vi "Session merge.vi"(7 "Loop Data":T1={"Persistent"={"Last file"=path "", "Last user"="", "Users"=[]}, "Temp handle"={"Connected"=FALSE, "Temp ctrl"={"Gain (P)"=0.0, "Reset (I)"=0.0, "Rate (D)"=0.0, "Stabilization rate"=0.0, "Stabilization delta"=0.0, "Type"=enum."Lake Shore 325", "Custom temp ctrl"={"VISA resource name"=""}, "Lakeshore 325"={"VISA name"="", "Loop"=0, "Heater Range"=1, "Heater Resistance"=0, "Sample sensor"=0, "Fast sensor"=0, "Slow sensor"=0}, "Lakeshore 331"={"VISA name"="", "Loop"=1, "Heater Range"=0, "Sample sensor"=0, "Fast sensor"=0, "Slow sensor"=0}, "Lakeshore 332"={"VISA name"="", "Loop"=1, "Heater Range"=0, "Sample sensor"=0, "Fast sensor"=0, "Slow sensor"=0}, "Lakeshore 335"={"VISA name"="", "Loop"=1, "Sample sensor"=0, "Fast sensor"=0, "Slow sensor"=0}}}, "Paths"={"Manual"=path "", "Settings"=path "", "Persistent"=path "", "Work dir."=path ""}, "Settings"={"MFIA"={"Address"="", "Use compensation"=FALSE, "Shut down gracefully"=FALSE}, "Temp ctrl"={"Gain (P)"=0.0, "Reset (I)"=0.0, "Rate (D)"=0.0, "Stabilization rate"=0.0, "Stabilization delta"=0.0, "Type"=enum."Lake Shore 325", "Custom temp ctrl"={"VISA resource name"=""}, "Lakeshore 325"={"VISA name"="", "Loop"=0, "Heater Range"=1, "Heater Resistance"=0, "Sample sensor"=0, "Fast sensor"=0, "Slow sensor"=0}, "Lakeshore 331"={"VISA name"="", "Loop"=1, "Heater Range"=0, "Sample sensor"=0, "Fast sensor"=0, "Slow sensor"=0}, "Lakeshore 332"={"VISA name"="", "Loop"=1, "Heater Range"=0, "Sample sensor"=0, "Fast sensor"=0, "Slow sensor"=0}, "Lakeshore 335"={"VISA name"="", "Loop"=1, "Sample sensor"=0, "Fast sensor"=0, "Slow sensor"=0}}, "Source-meter"={"Type"=enum."Custom", "Custom source-meter"={"VISA resource name"=""}, "Keithley 2600"={"VISA name"=""}}, "Other"={"Enable OriginLab"=FALSE, "Reader mode"=FALSE, "Auto-save"=FALSE}, "Defaults"={"IV properties"={"T"=300.0, "Vstart"=-0.5, "Vstop"=0.5, "Vpoints"=10.0, "Settling"=0.01, "I limit"=0.1, "Log mapping"=FALSE, "Averaging"=0.0}, "CV properties"={"T"=0.0, "Vstart"=-0.5, "Vstop"=0.5, "Vpoints"=10.0, "Precision"=enum."Normal", "Test signal"=0.01, "Auto I range"=FALSE, "Test frequency"=1000000.0, "I range"=-2.0, "V range"=10.0, "Log mapping"=FALSE, "Rel perm"=0.0, "Area"=0.0}, "DLTS properties"={"Tstart"=100.0, "Instant start"=FALSE, "Tstop"=300.0, "T rate"=5.0, "Test signal"=0.1, "Test frequency"=1000000.0, "Bandwidth"=5000.0, "Averaging"=10.0, "Vbias"=-2.0, "Vpulse"=-1.0, "pulse length"=0.001, "Pulse 2"=FALSE, "Vpulse 2"=0.0, "pulse length 2"=0.0, "I range"=-2.0, "V range"=10.0, "Emission rate"=[], "Sampling rate"=107142.859375, "Acq. delay"=0.0002}, "LDLTS properties"={"T"=0.0, "Test signal"=0.0, "Test frequency"=0.0, "Bandwidth"=0.0, "Averaging"=0.0, "Vbias"=0.0, "Vpulse"=0.0, "pulse length"=0.0, "Pulse 2"=FALSE, "Vpulse 2"=0.0, "pulse length 2"=0.0, "I range"=-2.0, "V range"=10.0, "Sampling rate"=0.0, "Acq. delay"=0.0, "Sampling time"=0.0}}}, "Software version"=0.0, "MFIA handle"={"ziHandle"={"handleValid"=FALSE, "Conn"=0, "Path Prefix"="", "Handle"=0, "Connected"=FALSE, "Clockbase(s)"=0.0}, "Selected device"="", "ziModHandle"={"handleValid"=FALSE, "Conn"=0, "ModHandle"=0, "moduleID"="", "Path Prefix"=""}}, "Source-meter handle"={"Connected"=FALSE, "Source-meter"={"Type"=enum."Keithley 2600", "Custom source-meter"={"VISA resource name"=""}, "Keithley 2600"={"VISA name"=""}}}} {"MFIA handle"."ziModHandle"."ModHandle" format="0x%08x"; "MFIA handle"."ziModHandle"."Conn" format="0x%08x"; "MFIA handle"."ziHandle"."Handle" format="0x%08x"; "MFIA handle"."ziHandle"."Conn" format="0x%08x"; "Settings"."Defaults"."LDLTS properties"."V range" items=["10mV"=0.01, "100mV"=0.1, "1V"=1.0, "10V"=10.0]; "Settings"."Defaults"."LDLTS properties"."I range" items=["100nA"=-7.0, "1µA"=-6.0, "10µA"=-5.0, "100µA"=-4.0, "1mA"=-3.0, "10mA"=-2.0]; "Settings"."Defaults"."DLTS properties"."V range" items=["10mV"=0.01, "100mV"=0.1, "1V"=1.0, "10V"=10.0]; "Settings"."Defaults"."DLTS properties"."I range" items=["10mV"=0.01, "100mV"=0.1, "1V"=1.0, "10V"=10.0]; "Settings"."Defaults"."CV properties"."V range" items=["10mV"=0.01, "100mV"=0.1, "1V"=1.0, "10V"=10.0]; "Settings"."Defaults"."CV properties"."I range" items=["100nA"=-7.0, "1µA"=-6.0, "10µA"=-5.0, "100µA"=-4.0, "1mA"=-3.0, "10mA"=-2.0]; "Settings"."Defaults"."IV properties"."Settling" min=0.0 max=65535.0; "Settings"."Temp ctrl"."Lakeshore 335"."Slow sensor" items=["A", "B"]; "Settings"."Temp ctrl"."Lakeshore 335"."Fast sensor" items=["A", "B"]; "Settings"."Temp ctrl"."Lakeshore 335"."Sample sensor" items=["A", "B"]; "Settings"."Temp ctrl"."Lakeshore 335"."Loop" items=["Loop 1"=1, "Loop 2"=2]; "Settings"."Temp ctrl"."Lakeshore 332"."Slow sensor" items=["A", "B"]; "Settings"."Temp ctrl"."Lakeshore 332"."Fast sensor" items=["A", "B"]; "Settings"."Temp ctrl"."Lakeshore 332"."Sample sensor" items=["A", "B"]; "Settings"."Temp ctrl"."Lakeshore 332"."Heater Range" items=["Off", "Low (0.5W)", "Med (5W)", "High (50W)"]; "Settings"."Temp ctrl"."Lakeshore 332"."Loop" items=["Loop 1", "Loop 2"]; "Settings"."Temp ctrl"."Lakeshore 331"."Slow sensor" items=["A", "B"]; "Settings"."Temp ctrl"."Lakeshore 331"."Fast sensor" items=["A", "B"]; "Settings"."Temp ctrl"."Lakeshore 331"."Sample sensor" items=["A", "B"]; "Settings"."Temp ctrl"."Lakeshore 331"."Heater Range" items=["Off", "Low (0.5W)", "Med (5W)", "High (50W)"]; "Settings"."Temp ctrl"."Lakeshore 331"."Loop" items=["Loop 1", "Loop 2"]; "Settings"."Temp ctrl"."Lakeshore 325"."Slow sensor" items=["A", "B"]; "Settings"."Temp ctrl"."Lakeshore 325"."Fast sensor" items=["A", "B"]; "Settings"."Temp ctrl"."Lakeshore 325"."Sample sensor" items=["A", "B"]; "Settings"."Temp ctrl"."Lakeshore 325"."Heater Resistance" items=["25 Ohm"=1, "50 Ohm"=2]; "Settings"."Temp ctrl"."Lakeshore 325"."Heater Range" items=["Off", "Low (loop 1) or On (loop 2)", "High (loop 1)"]; "Settings"."Temp ctrl"."Lakeshore 325"."Loop" items=["Loop 1"=1, "Loop 2"=2]; "Temp handle"."Temp ctrl"."Lakeshore 335"."Slow sensor" items=["A", "B"]; "Temp handle"."Temp ctrl"."Lakeshore 335"."Fast sensor" items=["A", "B"]; "Temp handle"."Temp ctrl"."Lakeshore 335"."Sample sensor" items=["A", "B"]; "Temp handle"."Temp ctrl"."Lakeshore 335"."Loop" items=["Loop 1"=1, "Loop 2"=2]; "Temp handle"."Temp ctrl"."Lakeshore 332"."Slow sensor" items=["A", "B"]; "Temp handle"."Temp ctrl"."Lakeshore 332"."Fast sensor" items=["A", "B"]; "Temp handle"."Temp ctrl"."Lakeshore 332"."Sample sensor" items=["A", "B"]; "Temp handle"."Temp ctrl"."Lakeshore 332"."Heater Range" items=["Off", "Low (0.5W)", "Med (5W)", "High (50W)"]; "Temp handle"."Temp ctrl"."Lakeshore 332"."Loop" items=["Loop 1", "Loop 2"]; "Temp handle"."Temp ctrl"."Lakeshore 331"."Slow sensor" items=["A", "B"]; "Temp handle"."Temp ctrl"."Lakeshore 331"."Fast sensor" items=["A", "B"]; "Temp handle"."Temp ctrl"."Lakeshore 331"."Sample sensor" items=["A", "B"]; "Temp handle"."Temp ctrl"."Lakeshore 331"."Heater Range" items=["Off", "Low (0.5W)", "Med (5W)", "High (50W)"]; "Temp handle"."Temp ctrl"."Lakeshore 331"."Loop" items=["Loop 1", "Loop 2"]; "Temp handle"."Temp ctrl"."Lakeshore 325"."Slow sensor" items=["A", "B"]; "Temp handle"."Temp ctrl"."Lakeshore 325"."Fast sensor" items=["A", "B"]; "Temp handle"."Temp ctrl"."Lakeshore 325"."Sample sensor" items=["A", "B"]; "Temp handle"."Temp ctrl"."Lakeshore 325"."Heater Resistance" items=["25 Ohm"=1, "50 Ohm"=2]; "Temp handle"."Temp ctrl"."Lakeshore 325"."Heater Range" items=["Off", "Low (loop 1) or On (loop 2)", "High (loop 1)"]; "Temp handle"."Temp ctrl"."Lakeshore 325"."Loop" items=["Loop 1"=1, "Loop 2"=2]}, 8 "Error In":errorcluster, 9 "Workspace":path, 10 "Index In":T20 {"IV"."IV properties"."Settling" min=0.0 max=65535.0; "CV"."CV properties"."V range" items=["10mV"=0.01, "100mV"=0.1, "1V"=1.0, "10V"=10.0]; "CV"."CV properties"."I range" items=["100nA"=-7.0, "1µA"=-6.0, "10µA"=-5.0, "100µA"=-4.0, "1mA"=-3.0, "10mA"=-2.0]; "LDLTS"."LDLTS properties"."V range" items=["10mV"=0.01, "100mV"=0.1, "1V"=1.0, "10V"=10.0]; "LDLTS"."LDLTS properties"."I range" items=["100nA"=-7.0, "1µA"=-6.0, "10µA"=-5.0, "100µA"=-4.0, "1mA"=-3.0, "10mA"=-2.0]; "Conv DLTS"."DLTS properties"."V range" items=["10mV"=0.01, "100mV"=0.1, "1V"=1.0, "10V"=10.0]; "Conv DLTS"."DLTS properties"."I range" items=["10mV"=0.01, "100mV"=0.1, "1V"=1.0, "10V"=10.0]}, 11 "Session properties in":T25) -> (0 "Error Out":errorcluster, 1 "Imported measurements count":i32, 2 "Index Out":T20 {"IV"."IV properties"."Settling" min=0.0 max=65535.0; "CV"."CV properties"."V range" items=["10mV"=0.01, "100mV"=0.1, "1V"=1.0, "10V"=10.0]; "CV"."CV properties"."I range" items=["100nA"=-7.0, "1µA"=-6.0, "10µA"=-5.0, "100µA"=-4.0, "1mA"=-3.0, "10mA"=-2.0]; "LDLTS"."LDLTS properties"."V range" items=["10mV"=0.01, "100mV"=0.1, "1V"=1.0, "10V"=10.0]; "LDLTS"."LDLTS properties"."I range" items=["100nA"=-7.0, "1µA"=-6.0, "10µA"=-5.0, "100µA"=-4.0, "1mA"=-3.0, "10mA"=-2.0]; "Conv DLTS"."DLTS properties"."V range" items=["10mV"=0.01, "100mV"=0.1, "1V"=1.0, "10V"=10.0]; "Conv DLTS"."DLTS properties"."I range" items=["10mV"=0.01, "100mV"=0.1, "1V"=1.0, "10V"=10.0]}, 3 "Session properties out":T25)   [LabVIEW 2019]
doc: "Displays information about a session"
uses:
  Type defs/Session properties Type Def.ctl
  Type defs/Session internal index Type Def.ctl
  Type defs/IV measurement Type Def.ctl
  Type defs/IV properties Type Def.ctl
  Type defs/CV measurement Type Def.ctl
  Type defs/CV properties Type Def.ctl
  Type defs/LDLTS measurement Type Def.ctl
  Type defs/LDLTS properties Type Def.ctl
  Type defs/cDLTS measurement Type Def.ctl
  Type defs/DLTS properties Type Def.ctl
  Type defs/Loop data Type Def.ctl
  Type defs/Persistent Type Def.ctl
  Type defs/Temp handle Type Def.ctl
  Type defs/Temp ctrl Type Def.ctl
  Custom devices/Custom temp ctrl settings.ctl
  Type defs/Paths Type Def.ctl
  Type defs/Settings Type Def.ctl
  Type defs/Imps Type Def.ctl
  Type defs/Source-meter Type Def.ctl
  Custom devices/Custom source-meter settings.ctl
  Type defs/Other settings Type Def.ctl
  Type defs/MFIA handle Type Def.ctl
  <instrlib>/Zurich Instruments LabOne/Public/ziTypeHandle.ctl
  <instrlib>/Zurich Instruments LabOne/Public/Modules/ziTypeModHandle.ctl
  Type defs/Source-meter handle Type Def.ctl
  <instrlib>/Zurich Instruments LabOne/Zurich Instruments LabOne.lvlib
panel:
  in  "Listbox":i32[](listbox) caption="Select measurements to import (duplicates cannot be imported)"
  out "Comment 2":string caption="Comment"
  out "Session Name 2":string caption="You're importing:"
  in  "Restore comment":bool
  in  "Restore name":bool
  in  "Cancel":bool
  in  "Apply":bool
  in  "Comment 1":string caption="Comment of the primary session"
  in  "Session Name 1":string caption="into the current session named:"
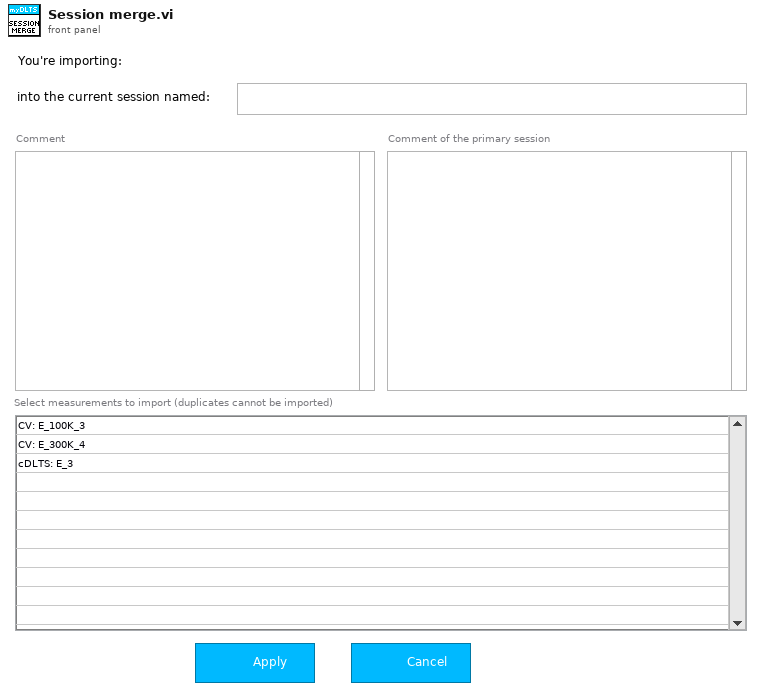
[diagram p1: front panel]
types:
  T1 = typedef "Loop data Type Def.ctl" = cluster{"Persistent":T2, "Temp handle":T3, "Paths":T6, "Settings":T7, "Software version":dbl, "MFIA handle":T16, "Source-meter handle":T19}
  T2 = typedef "Persistent Type Def.ctl" = cluster{"Last file":path, "Last user":string, "Users":cluster{"User":string, "Authors directory":path}[]}
  T3 = typedef "Temp handle Type Def.ctl" = cluster{"Connected":bool, "Temp ctrl":T4}
  T4 = typedef "Temp ctrl Type Def.ctl" = cluster{"Gain (P)":dbl, "Reset (I)":dbl, "Rate (D)":dbl, "Stabilization rate":dbl, "Stabilization delta":dbl, "Type":enum16{"Custom", "Lake Shore 325", "Lake Shore 331", "Lake Shore 332", "Lake Shore 335"}, "Custom temp ctrl":T5, "Lakeshore 325":cluster{"VISA name":refnum<visa-resource-name>, "Loop":u16, "Heater Range":u16, "Heater Resistance":u16, "Sample sensor":u16, "Fast sensor":u16, "Slow sensor":u16}, "Lakeshore 331":cluster{"VISA name":refnum<visa-resource-name>, "Loop":u16, "Heater Range":u16, "Sample sensor":u16, "Fast sensor":u16, "Slow sensor":u16}, "Lakeshore 332":cluster{"VISA name":refnum<visa-resource-name>, "Loop":u16, "Heater Range":u16, "Sample sensor":u16, "Fast sensor":u16, "Slow sensor":u16}, "Lakeshore 335":cluster{"VISA name":refnum<visa-resource-name>, "Loop":u16, "Sample sensor":u16, "Fast sensor":u16, "Slow sensor":u16}}
  T5 = typedef "Custom temp ctrl settings.ctl" = cluster{"VISA resource name":refnum<visa-resource-name>}
  T6 = typedef "Paths Type Def.ctl" = cluster{"Manual":path, "Settings":path, "Persistent":path, "Work dir.":path}
  T7 = typedef "Settings Type Def.ctl" = cluster{"MFIA":T8, "Temp ctrl":T4, "Source-meter":T9, "Other":T11, "Defaults":cluster{"IV properties":T12, "CV properties":T13, "DLTS properties":T14, "LDLTS properties":T15}}
  T8 = typedef "Imps Type Def.ctl" = cluster{"Address":string, "Use compensation":bool, "Shut down gracefully":bool}
  T9 = typedef "Source-meter Type Def.ctl" = cluster{"Type":enum16{"Custom", "Keithley 2600"}, "Custom source-meter":T10, "Keithley 2600":cluster{"VISA name":refnum<visa-resource-name>}}
  T10 = typedef "Custom source-meter settings.ctl" = cluster{"VISA resource name":refnum<visa-resource-name>}
  T11 = typedef "Other settings Type Def.ctl" = cluster{"Enable OriginLab":bool, "Reader mode":bool, "Auto-save":bool}
  T12 = typedef "IV properties Type Def.ctl" = cluster{"T":dbl[unit], "Vstart":dbl[unit], "Vstop":dbl[unit], "Vpoints":dbl, "Settling":dbl[unit], "I limit":dbl[unit], "Log mapping":bool, "Averaging":dbl}
  T13 = typedef "CV properties Type Def.ctl" = cluster{"T":dbl[unit], "Vstart":dbl[unit], "Vstop":dbl[unit], "Vpoints":dbl, "Precision":enum16{"Low (Fast)", "Normal", "High (Slow)"}, "Test signal":dbl[unit], "Auto I range":bool, "Test frequency":dbl[unit], "I range":dbl, "V range":dbl[unit], "Log mapping":bool, "Rel perm":dbl, "Area":dbl[unit]}
  T14 = typedef "DLTS properties Type Def.ctl" = cluster{"Tstart":dbl[unit], "Instant start":bool, "Tstop":dbl[unit], "T rate":dbl[unit], "Test signal":dbl[unit], "Test frequency":dbl[unit], "Bandwidth":dbl[unit], "Averaging":dbl, "Vbias":dbl[unit], "Vpulse":dbl[unit], "pulse length":dbl[unit], "Pulse 2":bool, "Vpulse 2":dbl[unit], "pulse length 2":dbl[unit], "I range":dbl, "V range":dbl[unit], "Emission rate":dbl[unit][], "Sampling rate":dbl[unit], "Acq. delay":dbl[unit]}
  T15 = typedef "LDLTS properties Type Def.ctl" = cluster{"T":dbl[unit], "Test signal":dbl[unit], "Test frequency":dbl[unit], "Bandwidth":dbl[unit], "Averaging":dbl, "Vbias":dbl[unit], "Vpulse":dbl[unit], "pulse length":dbl[unit], "Pulse 2":bool, "Vpulse 2":dbl[unit], "pulse length 2":dbl[unit], "I range":dbl, "V range":dbl[unit], "Sampling rate":dbl[unit], "Acq. delay":dbl[unit], "Sampling time":dbl[unit]}
  T16 = typedef "MFIA handle Type Def.ctl" = cluster{"ziHandle":T17, "Selected device":string, "ziModHandle":T18}
  T17 = typedef "Zurich Instruments LabOne.lvlib/ziTypeHandle.ctl" = cluster{"handleValid":bool, "Conn":u64, "Path Prefix":string, "Handle":u64, "Connected":bool, "Clockbase(s)":dbl}
  T18 = typedef "Zurich Instruments LabOne.lvlib/ziTypeModHandle.ctl" = cluster{"handleValid":bool, "Conn":u64, "ModHandle":u64, "moduleID":string, "Path Prefix":string}
  T19 = typedef "Source-meter handle Type Def.ctl" = cluster{"Connected":bool, "Source-meter":T9}
  T20 = typedef "Session internal index Type Def.ctl" = cluster{"IV":T21[], "CV":T22[], "LDLTS":T23[], "Conv DLTS":T24[]}
  T21 = typedef "IV measurement Type Def.ctl" = cluster{"Name":string, "Comment":string, "Time":timestamp, "Folder":path, "IV properties":T12, "GUID":string}
  T22 = typedef "CV measurement Type Def.ctl" = cluster{"Name":string, "Comment":string, "Time":timestamp, "Folder":path, "CV properties":T13, "GUID":string}
  T23 = typedef "LDLTS measurement Type Def.ctl" = cluster{"Name":string, "Comment":string, "Time":timestamp, "Folder":path, "LDLTS properties":T15, "GUID":string}
  T24 = typedef "cDLTS measurement Type Def.ctl" = cluster{"Name":string, "Comment":string, "Time":timestamp, "Folder":path, "DLTS properties":T14, "GUID":string}
  T25 = typedef "Session properties Type Def.ctl" = cluster{"Session name":string, "Comment":string, "User":string, "Software version":dbl, "Created":timestamp, "Modified":timestamp, "Binary":bool, "GUID":string}
  T26 = enum32{"Invalid", "Standard", "Closed", "Hidden", "Minimized", "Maximized"}
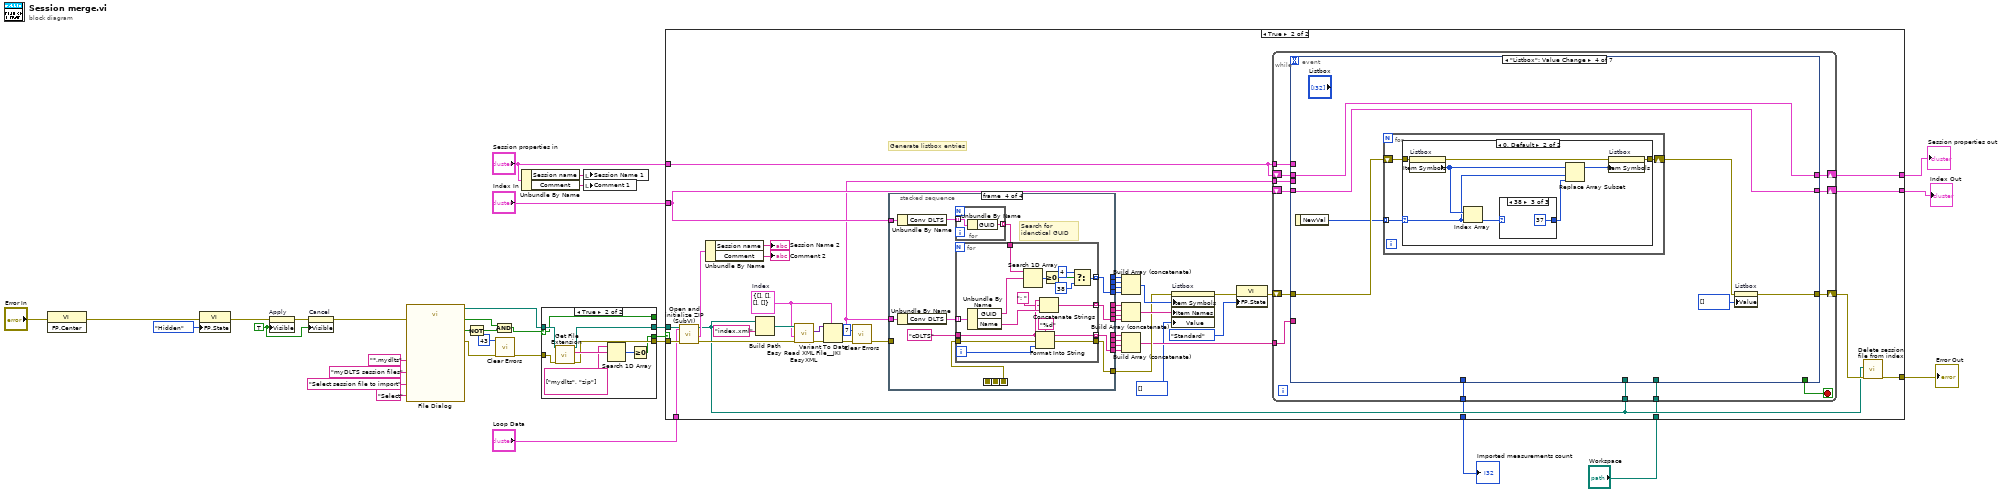
[diagram p0: block diagram]
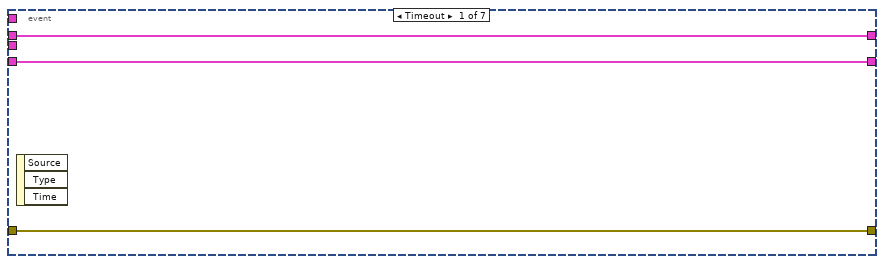
[diagram p3: hidden frame]
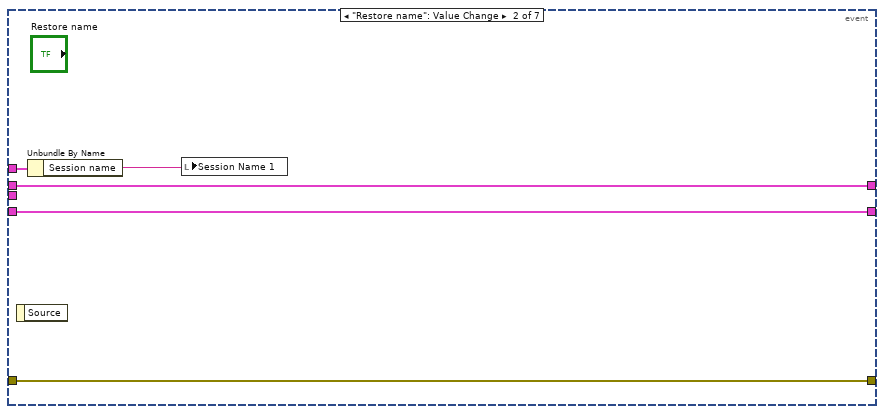
[diagram p4: hidden frame]
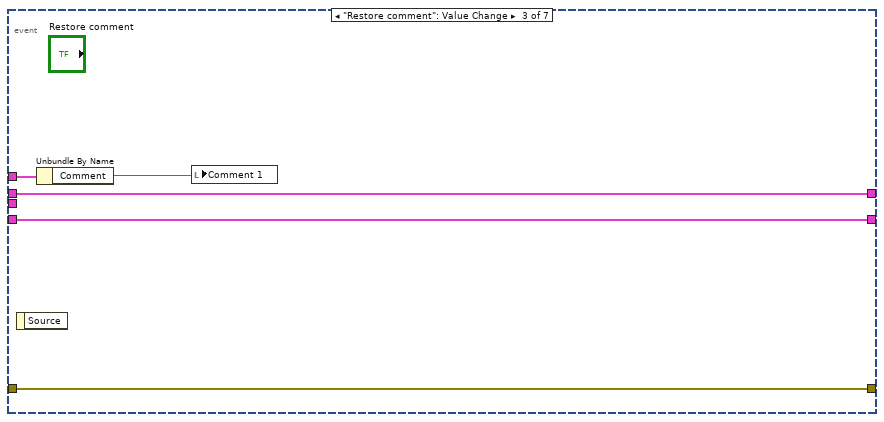
[diagram p5: hidden frame]
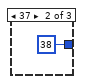
[diagram p8: hidden frame]
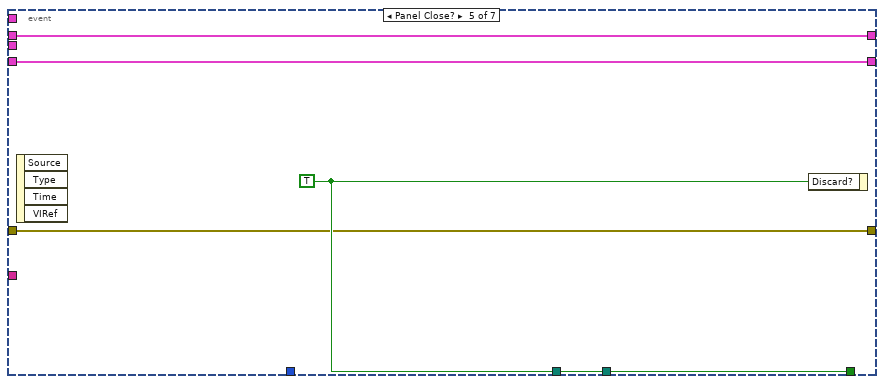
[diagram p9: hidden frame]
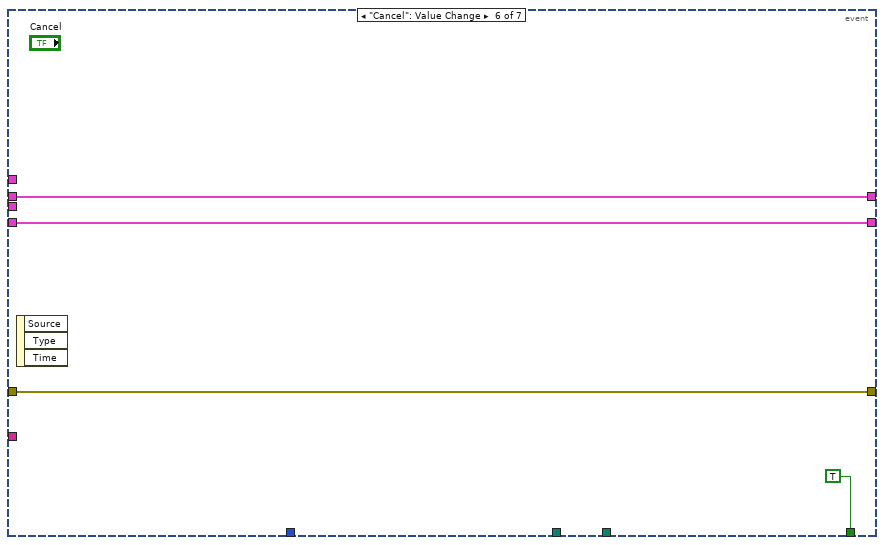
[diagram p10: hidden frame]
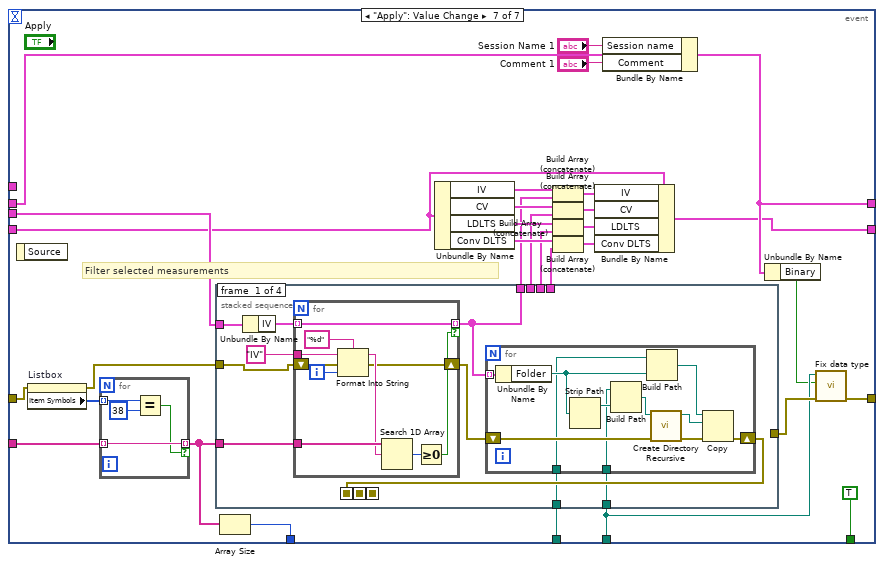
[diagram p11: hidden frame]
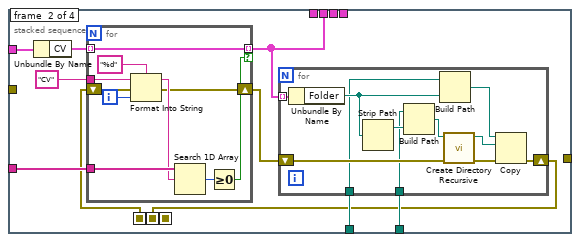
[diagram p12: hidden frame]
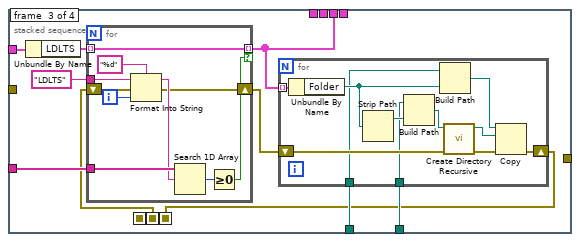
[diagram p13: hidden frame]
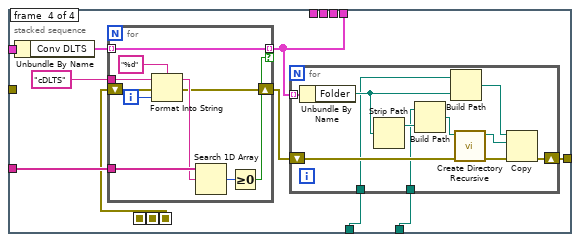
[diagram p14: hidden frame]
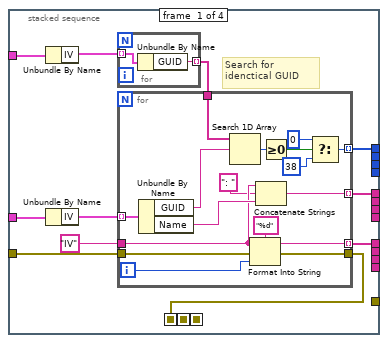
[diagram p15: hidden frame]
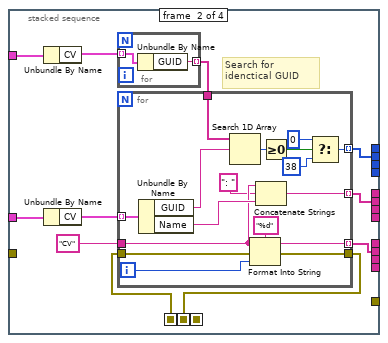
[diagram p16: hidden frame]
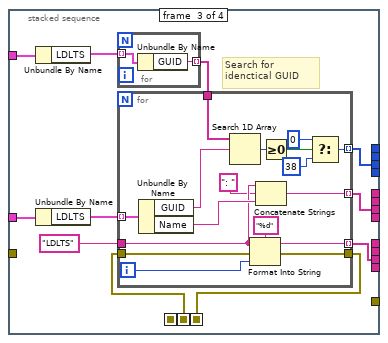
[diagram p17: hidden frame]
diagram:
  w30 = TRUE ("Visible")
  n1 = invoke class="VI" method="FP.Center"(error in="Error In") -> (error out=w1:errorcluster)  [unwired: 2 in, 2 out]
  n2 = property class="VI"(error in=w1, "FP.State"=T26."Hidden" ("Front Panel Window:State")) -> (error out=w2:errorcluster)  [unwired: 1 in, 1 out]
  n3 = property on="Apply" class="Bool"(error in=w2, "Visible"=w30) -> (error out=w31:errorcluster)  [unwired: 1 in, 1 out]
  n4 = property on="Cancel" class="Bool"(error in=w31, "Visible"=w30) -> (error out=w22:errorcluster)  [unwired: 1 in, 1 out]
  n5 = call "File Dialog"("prompt"="Select session file to import", "button label"="Select", "error in"=w22, "pattern (all files)"="*.mydlts", "pattern label"="myDLTS session files") -> ("selected path"=w21:path, "exists"=w18:bool, "cancelled"=w20:bool, "error out"=w5:errorcluster)  [unwired: 7 in]
  n6 = Not(x=w20) -> (.not. x?=w19:bool)
  n7 = And(x=w18, y=w19) -> (x .and. y?=w17:bool)
  n8 = call <vilib>:"Clear Errors.vi"("error in (no error)"=w5, "specific error code to clear (0: all)"=43) -> ("error out"=w4:errorcluster)  [unwired: 4 in, 1 out]
  n9 = Unbundle By Name("Session properties in") -> ("Session name"=w29:string, "Comment"=w28:string)
  n10 = case shown="True" w17 {
    selector: w17 -> [w33 w36]
    tunnel: w4 -> [w34 w43]
    tunnel: w21 -> [w35 w42]
    tunnel: [w35 w40] -> w25
    tunnel: [w34 w41] -> w26
    tunnel: [w33 w37] -> w27
    tunnel: [w33 w36] -> _
    frame False {
    }
    frame True {
      n11 = call <vilib>:"Get File Extension.vi"("error in (no error)"=w43, "file"=w42) -> ("error out"=w41:errorcluster, "lowercase file extension"=w44:string, "dup file"=w40:path)  [unwired: 5 in, 2 out]
      n12 = Search 1D Array(1D array=string[] ["mydlts", "zip"], element=w44) -> (index of element=w38:i32)  [unwired: 1 in]
      n13 = Greater Or Equal To 0?(x=w38) -> (x >= 0?=w37:bool)
    }
  }
  n14 = local write "Session Name 1"(w29) -> ()
  n15 = local write "Comment 1"(w28) -> ()
  n16 = case shown="True" w27 {
    tunnel: w26 -> [w46 w92]
    tunnel: w25 -> [_ w91]
    tunnel: "Loop Data" -> [_ w90]
    tunnel: "Index In" -> [w45 w62]
    tunnel: "Session properties in" -> [w47 w56]
    tunnel: [w47 w59] -> w11
    tunnel: [w46 w58] -> w10
    tunnel: "Workspace" -> [_ w54]
    tunnel: [w45 w53] -> w8
    tunnel: [_ w52] -> w7
    frame False {
    }
    frame True {
      w80 = T20 {"IV"=[], "CV"=[], "LDLTS"=[], "Conv DLTS"=[]}  # Index
      # "Generate listbox entries"
      n17 = call "Open and initialize ZIP (SubVI).vi"("Loop Data"=w90, "error in (no error)"=w92, "File to be opened"=w91) -> ("error out"=w79:errorcluster, "Session properties out"=w89:T25, "Workspace target"=w55:path)  [unwired: 5 in, 1 out]
      n18 = Unbundle By Name(w89) -> ("Session name"=→"Session Name 2":string, "Comment"=→"Comment 2":string)
      n19 = Build Path(base path=w55, name or relative path="index.xml") -> (appended path=w84:path)
      n20 = call <vilib>:"Easy Read XML File__JKI EasyXML.vi"("error in (no error)"=w79, "LabVIEW Data (Type)"=w80, "XML File Path"=w84) -> ("error out"=w85:errorcluster, "LabVIEW Data"=w83:variant)  [unwired: 6 in, 1 out]
      n21 = Variant To Data(error in=w85, type=w80, Variant=w83) -> (data=w57:T20, error out=w86:errorcluster)
      n22 = call <vilib>:"Clear Errors.vi"("error in (no error)"=w86, "specific error code to clear (0: all)"=7) -> ("error out"=w78:errorcluster)  [unwired: 4 in, 1 out]
      n23 = stacked-sequence {
        seq-local: [w310 _ _ _] -> [_ w342 _ _]
        seq-local: [_ w341 _ _] -> [_ _ w372 _]
        seq-local: [_ _ w371 _] -> [_ _ _ w402]
        tunnel: w78 -> [w315 _ _ _]
        tunnel: w57 -> [w318 w348 w378 w408]
        tunnel: w62 -> [w317 w347 w377 w407]
        tunnel: [w312 _ _ _] -> w77
        tunnel: [w311 _ _ _] -> w73
        tunnel: [w308 _ _ _] -> w69
        tunnel: [_ w340 _ _] -> w76
        tunnel: [_ w339 _ _] -> w72
        tunnel: [_ w338 _ _] -> w68
        tunnel: [_ _ w370 _] -> w75
        tunnel: [_ _ w369 _] -> w71
        tunnel: [_ _ w368 _] -> w67
        tunnel: [_ _ _ w401] -> w63
        tunnel: [_ _ _ w400] -> w66
        tunnel: [_ _ _ w399] -> w70
        tunnel: [_ _ _ w398] -> w74
        frame #0 {
          # "Search for idenctical GUID"
          n24 = Unbundle By Name(w317) -> ("IV"=w314:T21[])
          n25 = Unbundle By Name(w318) -> ("IV"=w316:T21[])
          n26 = for {
            tunnel: w314 -> [w320] mode=indexing
            tunnel: [w319] -> w313 mode=indexing
            n27 = Unbundle By Name(w320) -> ("GUID"=w319:string)
          }
          n28 = for {
            tunnel: w316 -> [w337] mode=indexing
            tunnel: w315 -> [w328]
            tunnel: w313 -> [w335]
            tunnel: [w321] -> w311 mode=indexing
            tunnel: [w330] -> w312 mode=indexing
            tunnel: [w327] -> w310
            tunnel: "IV" ("format string") -> [w323]
            tunnel: [w326] -> w308 mode=indexing
            i -> [w329]
            n29 = Unbundle By Name(w337) -> ("GUID"=w336:string, "Name"=w324:string)
            n30 = Search 1D Array(1D array=w335, element=w336) -> (index of element=w334:i32)  [unwired: 1 in]
            n31 = Format Into String(format string="%d", initial string=w323, error in=w328, w329) -> (resulting string=w326:string, error out=w327:errorcluster)
            n32 = Concatenate Strings(w323, ": " ("string"), w324) -> (w321:string)
            n33 = Greater Or Equal To 0?(x=w334) -> (x >= 0?=w333:bool)
            n34 = Select(t=0, s=w333, f=38 ("y")) -> (s? t:f=w330:i32)
          }
        }
        frame #1 {
          # "Search for idenctical GUID"
          n35 = Unbundle By Name(w347) -> ("CV"=w345:T22[])
          n36 = Unbundle By Name(w348) -> ("CV"=w346:T22[])
          n37 = for {
            tunnel: w345 -> [w350] mode=indexing
            tunnel: [w349] -> w344 mode=indexing
            n38 = Unbundle By Name(w350) -> ("GUID"=w349:string)
          }
          n39 = for {
            tunnel: w346 -> [w367] mode=indexing
            tunnel: w342 -> [w358]
            tunnel: w344 -> [w365]
            tunnel: [w351] -> w339 mode=indexing
            tunnel: [w360] -> w340 mode=indexing
            tunnel: [w357] -> w341
            tunnel: "CV" ("format string") -> [w353]
            tunnel: [w356] -> w338 mode=indexing
            i -> [w359]
            n40 = Unbundle By Name(w367) -> ("GUID"=w366:string, "Name"=w354:string)
            n41 = Search 1D Array(1D array=w365, element=w366) -> (index of element=w364:i32)  [unwired: 1 in]
            n42 = Format Into String(format string="%d", initial string=w353, error in=w358, w359) -> (resulting string=w356:string, error out=w357:errorcluster)
            n43 = Concatenate Strings(w353, ": " ("string"), w354) -> (w351:string)
            n44 = Greater Or Equal To 0?(x=w364) -> (x >= 0?=w363:bool)
            n45 = Select(t=0, s=w363, f=38 ("y")) -> (s? t:f=w360:i32)
          }
        }
        frame #2 {
          # "Search for idenctical GUID"
          n46 = Unbundle By Name(w377) -> ("LDLTS"=w375:T23[])
          n47 = Unbundle By Name(w378) -> ("LDLTS"=w376:T23[])
          n48 = for {
            tunnel: w375 -> [w380] mode=indexing
            tunnel: [w379] -> w374 mode=indexing
            n49 = Unbundle By Name(w380) -> ("GUID"=w379:string)
          }
          n50 = for {
            tunnel: w376 -> [w397] mode=indexing
            tunnel: w372 -> [w388]
            tunnel: w374 -> [w395]
            tunnel: [w381] -> w369 mode=indexing
            tunnel: [w390] -> w370 mode=indexing
            tunnel: [w387] -> w371
            tunnel: "LDLTS" ("format string") -> [w383]
            tunnel: [w386] -> w368 mode=indexing
            i -> [w389]
            n51 = Unbundle By Name(w397) -> ("GUID"=w396:string, "Name"=w384:string)
            n52 = Search 1D Array(1D array=w395, element=w396) -> (index of element=w394:i32)  [unwired: 1 in]
            n53 = Format Into String(format string="%d", initial string=w383, error in=w388, w389) -> (resulting string=w386:string, error out=w387:errorcluster)
            n54 = Concatenate Strings(w383, ": " ("string"), w384) -> (w381:string)
            n55 = Greater Or Equal To 0?(x=w394) -> (x >= 0?=w393:bool)
            n56 = Select(t=0, s=w393, f=38 ("y")) -> (s? t:f=w390:i32)
          }
        }
        frame #3 {
          # "Search for idenctical GUID"
          n57 = Unbundle By Name(w407) -> ("Conv DLTS"=w405:T24[])
          n58 = Unbundle By Name(w408) -> ("Conv DLTS"=w406:T24[])
          n59 = for {
            tunnel: w405 -> [w410] mode=indexing
            tunnel: [w409] -> w404 mode=indexing
            n60 = Unbundle By Name(w410) -> ("GUID"=w409:string)
          }
          n61 = for {
            tunnel: w406 -> [w427] mode=indexing
            tunnel: w402 -> [w418]
            tunnel: w404 -> [w425]
            tunnel: [w411] -> w399 mode=indexing
            tunnel: [w420] -> w398 mode=indexing
            tunnel: [w417] -> w401
            tunnel: "cDLTS" ("format string") -> [w413]
            tunnel: [w416] -> w400 mode=indexing
            i -> [w419]
            n62 = Unbundle By Name(w427) -> ("GUID"=w426:string, "Name"=w414:string)
            n63 = Search 1D Array(1D array=w425, element=w426) -> (index of element=w424:i32)  [unwired: 1 in]
            n64 = Format Into String(format string="%d", initial string=w413, error in=w418, w419) -> (resulting string=w416:string, error out=w417:errorcluster)
            n65 = Concatenate Strings(w413, ": " ("string"), w414) -> (w411:string)
            n66 = Greater Or Equal To 0?(x=w424) -> (x >= 0?=w423:bool)
            n67 = Select(t=4, s=w423, f=38 ("y")) -> (s? t:f=w420:i32)
          }
        }
      }
      n68 = Build Array (concatenate)(w77, w76, w75, w74) -> (w65:i32[])
      n69 = Build Array (concatenate)(w73, w72, w71, w70) -> (w64:string[])
      n70 = Build Array (concatenate)(w69, w68, w67, w66) -> (w61:string[])
      n71 = property on="Listbox" class="LstBox (strict)"(error in=w63, "Item Symbols"=w65, "Item Names"=w64, "Value"=i32[] [] ("Listbox")) -> (error out=w49:errorcluster)  [unwired: 1 in, 1 out]
      n72 = property class="VI"(error in=w49, "FP.State"=T26."Standard" ("Front Panel Window:State")) -> (error out=w50:errorcluster)  [unwired: 1 in, 1 out]
      n73 = while {
        shift-right: [w102] -> w59
        shift-left: w56 -> [w103]
        shift-right: [w101] -> w60
        shift-left: w50 -> [w104]
        tunnel: w56 -> [w100]
        tunnel: w61 -> [w98]
        tunnel: w57 -> [w97]
        tunnel: w55 -> [w96]
        tunnel: w54 -> [w95]
        shift-right: [w94] -> w53
        shift-left: w62 -> [w99]
        tunnel: [w93] -> w52
        stop <- w105 stop-if-true
        n74 = event shown="[3] \"Listbox\": Value Change" {
          selector: _ -> [_ _ _ _ _ _ _]
          dyn-events: _ -> [_ _ _ _ _ _ _]
          timeout: _ -> [_ _ _ _ _ _ _]
          tunnel: [_ _ _ _ w144 TRUE ("Discard?") TRUE ("Discard?")] -> w105
          tunnel: w104 -> [w107 w110 w115 w125 w142 w146 w175]
          tunnel: w103 -> [w108 w113 w118 w124 w143 w148 w155]
          tunnel: [w108 w113 w118 w124 w143 w148 w153] -> w102
          tunnel: [w107 w110 w115 w120 w142 w146 w157] -> w101
          tunnel: w100 -> [_ w112 w117 _ _ _ _]
          tunnel: w99 -> [w106 w109 w114 w123 w141 w145 w172]
          tunnel: w98 -> [_ _ _ _ _ _ w151]
          tunnel: w97 -> [_ _ _ _ _ _ w174]
          tunnel: w96 -> [_ _ _ _ _ _ w159]
          tunnel: w95 -> [_ _ _ _ _ _ w156]
          tunnel: [w106 w109 w114 w123 w141 w145 w152] -> w94
          tunnel: [_ _ _ _ _ _ w150] -> w93
          event Timeout {
            n75 = event-data() -> ()  [unwired: 1 in, 3 out]
          }
          event "Restore name": Value Change {
            n76 = event-data() -> ()  [unwired: 1 in, 1 out]
            n77 = Unbundle By Name(w112) -> ("Session name"=w111:string)
            n78 = local write "Session Name 1"(w111) -> ()
          }
          event "Restore comment": Value Change {
            n79 = event-data() -> ()  [unwired: 1 in, 1 out]
            n80 = Unbundle By Name(w117) -> ("Comment"=w116:string)
            n81 = local write "Comment 1"(w116) -> ()
          }
          event "Listbox": Value Change {
            n82 = event-data() -> ("NewVal"=w119:i32[])  [unwired: 1 in]
            n83 = for {
              shift-right: [w127] -> w121
              shift-left: w125 -> [w128]
              tunnel: w119 -> [w126] mode=indexing
              n84 = case shown="0, Default" w126 {
                selector: w126 -> [_ w136]
                tunnel: [w129 w131] -> w127
                tunnel: w128 -> [w129 w130]
                frame -1 {
                }
                frame 0, Default {
                  n85 = property on="Listbox" class="LstBox (strict)"(error in=w130) -> (error out=w132:errorcluster, "Item Symbols"=w137:i32[])  [unwired: 1 in, 1 out]
                  n86 = Index Array(array=w137, index=w136) -> (element=w135:i32)
                  n87 = case shown="38" w135 {
                    selector: w135 -> [w138 _ _]
                    tunnel: [w138 38 37] -> w134
                    frame 0, Default {
                    }
                    frame 37 {
                    }
                    frame 38 {
                    }
                  }
                  n88 = Replace Array Subset(array=w137, new element=w134, index=w136) -> (w133:i32[])
                  n89 = property on="Listbox" class="LstBox (strict)"(error in=w132, "Item Symbols"=w133) -> (error out=w131:errorcluster)  [unwired: 1 in, 1 out]
                }
              }
            }
            n90 = property on="Listbox" class="LstBox (strict)"(error in=w121, "Value"=i32[] [] ("Listbox")) -> (error out=w120:errorcluster)  [unwired: 1 in, 1 out]
          }
          event Panel Close? {
            w144 = TRUE ("Discard?")
            n91 = event-data() -> ()  [unwired: 1 in, 4 out]
            n92 = event-data("Discard?"=w144) -> ()  [unwired: 1 in, 1 out]
          }
          event "Cancel": Value Change {
            n93 = event-data() -> ()  [unwired: 1 in, 3 out]
          }
          event "Apply": Value Change {
            # "Filter selected measurements"
            n94 = event-data() -> ()  [unwired: 1 in, 1 out]
            n95 = property on="Listbox" class="LstBox (strict)"(error in=w175) -> (error out=w173:errorcluster, "Item Symbols"=w176:i32[])  [unwired: 1 in, 1 out]
            n96 = for {
              tunnel: w176 -> [w307] mode=indexing
              tunnel: [w305] -> w149 mode=indexing if=w304
              tunnel: w151 -> [w305] mode=indexing
              n97 = Equal?(x=w307, y=38) -> (x = y?=w304:bool)
            }
            n98 = stacked-sequence {
              seq-local: [w182 _ _ _] -> [_ w216 _ _]
              seq-local: [_ w211 _ _] -> [_ _ w247 _]
              seq-local: [_ _ w242 _] -> [_ _ _ w278]
              tunnel: w174 -> [w189 w220 w251 w282]
              tunnel: w149 -> [w186 w217 w248 w279]
              tunnel: w173 -> [w185 _ _ _]
              tunnel: [w184 _ _ _] -> w163
              tunnel: [_ w215 _ _] -> w162
              tunnel: [_ _ w246 _] -> w161
              tunnel: [_ _ _ w275] -> w160
              tunnel: w159 -> [w181 w213 w245 w277]
              tunnel: w156 -> [w180 w212 w244 w276]
              tunnel: [_ _ _ w273] -> w158
              frame #0 {
                n99 = Unbundle By Name(w189) -> ("IV"=w188:T21[])
                n100 = for {
                  tunnel: w188 -> [w201] mode=indexing
                  tunnel: "IV" ("format string") -> [w208]
                  tunnel: w186 -> [w210]
                  tunnel: [w201] -> w184 mode=indexing if=w203
                  shift-right: [w202] -> w183
                  shift-left: w185 -> [w206]
                  i -> [w207]
                  n101 = Format Into String(format string="%d", initial string=w208, error in=w206, w207) -> (resulting string=w205:string, error out=w202:errorcluster)
                  n102 = Search 1D Array(1D array=w210, element=w205) -> (index of element=w204:i32)  [unwired: 1 in]
                  n103 = Greater Or Equal To 0?(x=w204) -> (x >= 0?=w203:bool)
                }
                n104 = for {
                  shift-right: [w194] -> w182
                  shift-left: w183 -> [w193]
                  tunnel: w184 -> [w192] mode=indexing
                  tunnel: w181 -> [w191]
                  tunnel: w180 -> [w190]
                  n105 = Unbundle By Name(w192) -> ("Folder"=w195:path)
                  n106 = Strip Path(path=w195) -> (stripped path=w199:path)  [unwired: 1 out]
                  n107 = Build Path(base path=w190, name or relative path=w199) -> (appended path=w198:path)
                  n108 = Build Path(base path=w191, name or relative path=w195) -> (appended path=w200:path)
                  n109 = call <vilib>:"Create Directory Recursive.vi"("error in (no error)"=w193, "directory"=w198) -> ("error out"=w196:errorcluster, "directory copy"=w197:path)  [unwired: 3 in, 1 out]
                  n110 = Copy(8:w196, 10:w197, 11:w200) -> (0:w194:errorcluster)  [unwired: 2 in, 2 out]
                }
              }
              frame #1 {
                n111 = Unbundle By Name(w220) -> ("CV"=w219:T22[])
                n112 = for {
                  tunnel: w219 -> [w234] mode=indexing
                  tunnel: "CV" ("format string") -> [w239]
                  tunnel: w217 -> [w241]
                  tunnel: [w234] -> w215 mode=indexing if=w233
                  shift-right: [w232] -> w214
                  shift-left: w216 -> [w237]
                  i -> [w238]
                  n113 = Format Into String(format string="%d", initial string=w239, error in=w237, w238) -> (resulting string=w236:string, error out=w232:errorcluster)
                  n114 = Search 1D Array(1D array=w241, element=w236) -> (index of element=w235:i32)  [unwired: 1 in]
                  n115 = Greater Or Equal To 0?(x=w235) -> (x >= 0?=w233:bool)
                }
                n116 = for {
                  shift-right: [w221] -> w211
                  shift-left: w214 -> [w225]
                  tunnel: w215 -> [w224] mode=indexing
                  tunnel: w213 -> [w223]
                  tunnel: w212 -> [w222]
                  n117 = Unbundle By Name(w224) -> ("Folder"=w226:path)
                  n118 = Strip Path(path=w226) -> (stripped path=w230:path)  [unwired: 1 out]
                  n119 = Build Path(base path=w222, name or relative path=w230) -> (appended path=w229:path)
                  n120 = Build Path(base path=w223, name or relative path=w226) -> (appended path=w231:path)
                  n121 = call <vilib>:"Create Directory Recursive.vi"("error in (no error)"=w225, "directory"=w229) -> ("error out"=w227:errorcluster, "directory copy"=w228:path)  [unwired: 3 in, 1 out]
                  n122 = Copy(8:w227, 10:w228, 11:w231) -> (0:w221:errorcluster)  [unwired: 2 in, 2 out]
                }
              }
              frame #2 {
                n123 = Unbundle By Name(w251) -> ("LDLTS"=w250:T23[])
                n124 = for {
                  tunnel: w250 -> [w265] mode=indexing
                  tunnel: "LDLTS" ("format string") -> [w270]
                  tunnel: w248 -> [w272]
                  tunnel: [w265] -> w246 mode=indexing if=w264
                  shift-right: [w263] -> w243
                  shift-left: w247 -> [w268]
                  i -> [w269]
                  n125 = Format Into String(format string="%d", initial string=w270, error in=w268, w269) -> (resulting string=w267:string, error out=w263:errorcluster)
                  n126 = Search 1D Array(1D array=w272, element=w267) -> (index of element=w266:i32)  [unwired: 1 in]
                  n127 = Greater Or Equal To 0?(x=w266) -> (x >= 0?=w264:bool)
                }
                n128 = for {
                  shift-right: [w256] -> w242
                  shift-left: w243 -> [w255]
                  tunnel: w246 -> [w254] mode=indexing
                  tunnel: w245 -> [w253]
                  tunnel: w244 -> [w252]
                  n129 = Unbundle By Name(w254) -> ("Folder"=w257:path)
                  n130 = Strip Path(path=w257) -> (stripped path=w261:path)  [unwired: 1 out]
                  n131 = Build Path(base path=w252, name or relative path=w261) -> (appended path=w260:path)
                  n132 = Build Path(base path=w253, name or relative path=w257) -> (appended path=w262:path)
                  n133 = call <vilib>:"Create Directory Recursive.vi"("error in (no error)"=w255, "directory"=w260) -> ("error out"=w258:errorcluster, "directory copy"=w259:path)  [unwired: 3 in, 1 out]
                  n134 = Copy(8:w258, 10:w259, 11:w262) -> (0:w256:errorcluster)  [unwired: 2 in, 2 out]
                }
              }
              frame #3 {
                n135 = Unbundle By Name(w282) -> ("Conv DLTS"=w281:T24[])
                n136 = for {
                  tunnel: w281 -> [w296] mode=indexing
                  tunnel: "cDLTS" ("format string") -> [w301]
                  tunnel: w279 -> [w303]
                  tunnel: [w296] -> w275 mode=indexing if=w295
                  shift-right: [w294] -> w274
                  shift-left: w278 -> [w299]
                  i -> [w300]
                  n137 = Format Into String(format string="%d", initial string=w301, error in=w299, w300) -> (resulting string=w298:string, error out=w294:errorcluster)
                  n138 = Search 1D Array(1D array=w303, element=w298) -> (index of element=w297:i32)  [unwired: 1 in]
                  n139 = Greater Or Equal To 0?(x=w297) -> (x >= 0?=w295:bool)
                }
                n140 = for {
                  shift-right: [w287] -> w273
                  shift-left: w274 -> [w286]
                  tunnel: w275 -> [w285] mode=indexing
                  tunnel: w277 -> [w284]
                  tunnel: w276 -> [w283]
                  n141 = Unbundle By Name(w285) -> ("Folder"=w288:path)
                  n142 = Strip Path(path=w288) -> (stripped path=w292:path)  [unwired: 1 out]
                  n143 = Build Path(base path=w283, name or relative path=w292) -> (appended path=w291:path)
                  n144 = Build Path(base path=w284, name or relative path=w288) -> (appended path=w293:path)
                  n145 = call <vilib>:"Create Directory Recursive.vi"("error in (no error)"=w286, "directory"=w291) -> ("error out"=w289:errorcluster, "directory copy"=w290:path)  [unwired: 3 in, 1 out]
                  n146 = Copy(8:w289, 10:w290, 11:w293) -> (0:w287:errorcluster)  [unwired: 2 in, 2 out]
                }
              }
            }
            n147 = Array Size(array=w149) -> (size(s)=w150:i32)
            n148 = Unbundle By Name(w172) -> ("IV"=w170:T21[], "CV"=w169:T22[], "LDLTS"=w167:T23[], "Conv DLTS"=w165:T24[])
            n149 = Build Array (concatenate)(w170, w163) -> (w171:T21[])
            n150 = Build Array (concatenate)(w169, w162) -> (w168:T22[])
            n151 = Build Array (concatenate)(w167, w161) -> (w166:T23[])
            n152 = Build Array (concatenate)(w165, w160) -> (w164:T24[])
            n153 = Bundle By Name(cluster=w172, "IV"=w171, "CV"=w168, "LDLTS"=w166, "Conv DLTS"=w164) -> (w152:T20)
            n154 = Bundle By Name(cluster=w155, "Session name"="Session Name 1", "Comment"="Comment 1") -> (w153:T25)
            n155 = Unbundle By Name(w153) -> ("Binary"=w154:bool)
            n156 = call "Fix data type.vi"("error in (no error)"=w158, "Binary?"=w154, "Workspace"=w156) -> ("error out"=w157:errorcluster)  [unwired: 8 in]
          }
        }
      }
      n157 = call "Delete session file from index.vi"("Workspace path"=w55, "error in (no error)"=w60) -> ("error out"=w58:errorcluster)  [unwired: 7 in, 1 out]
    }
  }
  "Error Out" <- w10
  "Session properties out" <- w11
  "Index Out" <- w8
  "Imported measurements count" <- w7
